vi "Configure Digital Filter.vi"(0 "VISA resource name":refnum<visa-resource-name>, 1 "Enable Digital Filter (F: Disable)":bool, 2 "Filter Count (10)":i32=10 min=1 max=100, 5 "Digital Filter Type (0: Repeating)":u16(ring) items=["Repeating", "Moving"], 11 "error in (no error)":errorcluster) -> (4 "VISA resource name out":refnum<visa-resource-name>, 15 "error out":errorcluster)   [LabVIEW 2016, in "Keithley 6517.lvlib"]
doc: "Configures the digital filter for model 6514.\n\n<B>Note:</B>\nThis VI is ONLY compatible with <B>model 6514</B>. Running this VI with any other model will result in an error."
uses:
  <instrlib>/Keithley 6517/Keithley 6517.lvlib
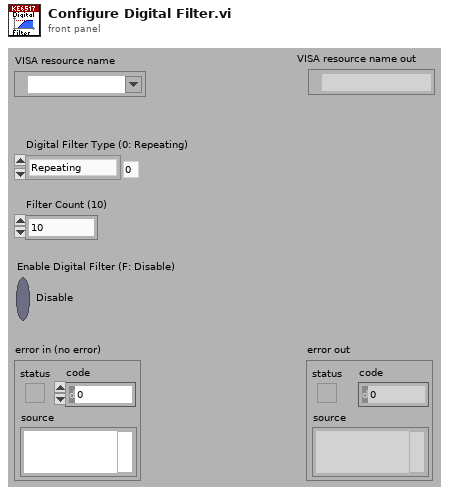
[diagram p1: front panel]
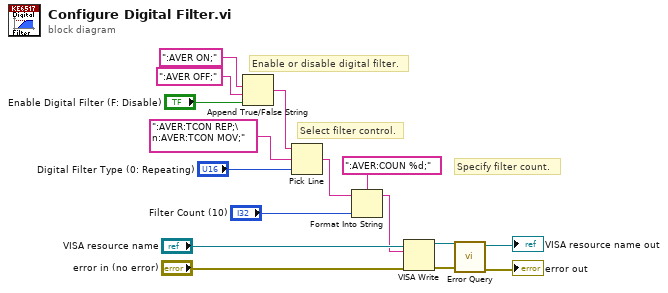
[diagram p0: block diagram]
diagram:
  # "Specify filter count."
  # "Select filter control."
  # "Enable or disable digital filter."
  n1 = Append True/False String(1:"Enable Digital Filter (F: Disable)", 2:":AVER OFF;" ("false string"), 3:":AVER ON;" ("true string")) -> (0:w2:string)  [unwired: 1 in]
  n2 = Pick Line(string ("")=w2, multi-line string=":AVER:TCON REP;\n:AVER:TCON MOV;", line index="Digital Filter Type (0: Repeating)") -> (output string=w4:string)
  n3 = Format Into String(format string=":AVER:COUN %d;", initial string=w4, "Filter Count (10)") -> (resulting string=w5:string)  [unwired: 1 in, 1 out]
  n4 = VISA Write(VISA resource name="VISA resource name", write buffer=w5, error in (no error)="error in (no error)") -> (VISA resource name out=w10:refnum<visa-resource-name>, error out=w11:errorcluster)  [unwired: 1 out]
  n5 = call <instrlib>:"Error Query.vi"("error in (no error)"=w11, "VISA resource name"=w10) -> ("error out"=→"error out":errorcluster, "VISA resource name out"=→"VISA resource name out":refnum<visa-resource-name>)  [unwired: 6 in, 2 out]
